vi "Sub_Set_Voltage_SweepOutput.vi"(0 "AgB29xxLib.IAgB29xx2":refnum<k7>, 5 "i":u32=5, 9 "Mode":i32(ring)=2 items=["AgB29xxTransientCurrentVoltageModeFixed", "AgB29xxTransientCurrentVoltageModeList", "AgB29xxTransientCurrentVoltageModeSweep"], 11 "error in (no error)":errorcluster, 12 "Start":dbl=-5.0, 13 "Stop":dbl=5.0, 14 "Sweep Points":u32=11) -> (4 "AgB29xxLib.IAgB29xx2 2":refnum<k7>, 15 "error out":errorcluster)   [LabVIEW 2009]
panel:
  # "Sub VI: Set Voltage Sweep Output"
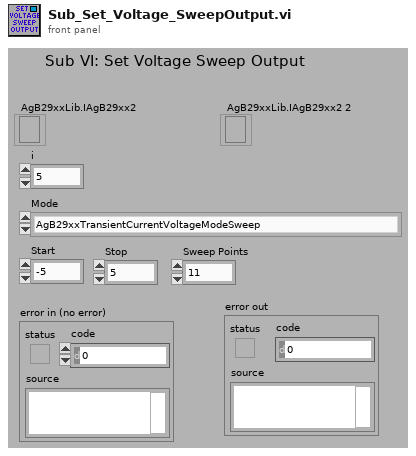
[diagram p1: front panel]
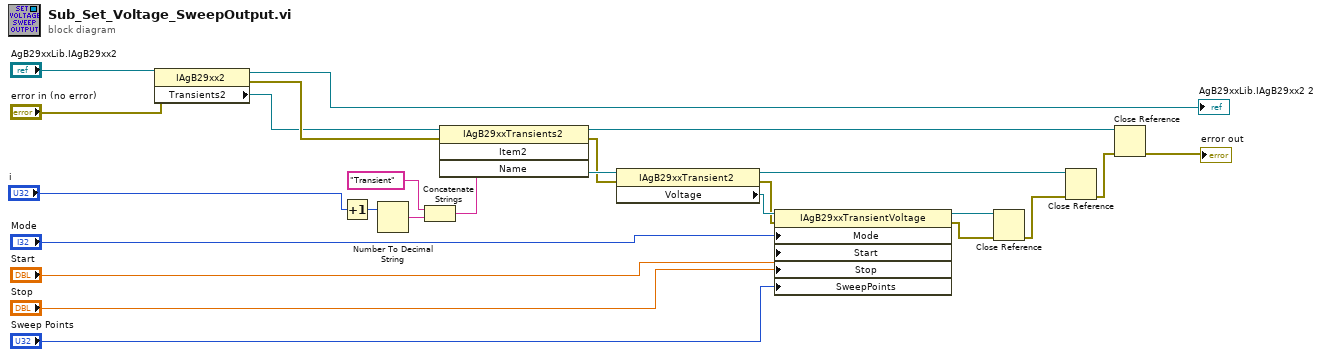
[diagram p0: block diagram]
diagram:
  n1 = property class="IAgB29xx2"(reference="AgB29xxLib.IAgB29xx2", error in="error in (no error)") -> (reference out=→"AgB29xxLib.IAgB29xx2 2":refnum<k7>, error out=w17:errorcluster, "Transients2"=w16:refnum<k7>)
  n2 = Increment(x="i") -> (x+1=w14:u32)
  n3 = Number To Decimal String(number=w14) -> (decimal integer string=w13:string)  [unwired: 1 in]
  n4 = Concatenate Strings("Transient" ("string"), w13) -> (w11:string)
  n5 = invoke class="IAgB29xxTransients2" method="Item2"(reference=w16, error in=w17, "Name"=w11) -> (reference out=w7:refnum<k7>, error out=w10:errorcluster, "Item2"=w15:refnum<k7>)  [unwired: 1 in, 1 out]
  n6 = property class="IAgB29xxTransient2"(reference=w15, error in=w10) -> (reference out=w9:refnum<k7>, error out=w5:errorcluster, "Voltage"=w6:refnum<k7>)
  n7 = property class="IAgB29xxTransientVoltage"(reference=w6, error in=w5, "Mode"="Mode", "Start"="Start", "Stop"="Stop", "SweepPoints"="Sweep Points") -> (reference out=w3:refnum<k7>, error out=w2:errorcluster)
  n8 = Close Reference(reference=w3, error in (no error)=w2) -> (error out=w4:errorcluster)
  n9 = Close Reference(reference=w9, error in (no error)=w4) -> (error out=w8:errorcluster)
  n10 = Close Reference(reference=w7, error in (no error)=w8) -> (error out=→"error out":errorcluster)
